vi "Settings Dialog.vi"(8 "error in (no error)":T5 caption="entrée d'erreur (pas d'erreur)", 11 "Paramètres en entrée":T1={"Configuration du matériel"={"Refnum de matériel <À remplacer>"="", "Type de signal <À remplacer>"=enum."Sine Wave", "Choix de la longueur d'onde"=500.0, "Nom du périphérique"="Dev1", "Choix mode"=FALSE}, "Configuration de l'enregistrement"={"Chemin de base du fichier journal"=path "", "Référence de fichier TDMS"=refnum}, "Commande numérique"=0.0}) -> (0 "error out":T5 caption="sortie d'erreur", 1 "Annulation ?":bool, 2 "Actualisation de l'IU requise ?":bool, 3 "Paramètres en sortie":T1={"Configuration du matériel"={"Refnum de matériel <À remplacer>"="", "Type de signal <À remplacer>"=enum."Sine Wave", "Choix de la longueur d'onde"=500.0, "Nom du périphérique"="Dev1", "Choix mode"=FALSE}, "Configuration de l'enregistrement"={"Chemin de base du fichier journal"=path "", "Référence de fichier TDMS"=refnum}, "Commande numérique"=0.0})   [LabVIEW 2018, in "Settings.lvlib"]
doc: "Boîte de dialogue permettant de sélectionner les paramètres spécifiés par l'utilisateur."
uses:
  Settings.lvlib
  Settings.ctl
  Acquisition/Hardware Configuration.ctl
  Acquisition/Signal Type.ctl
  Logging/Logging Configuration.ctl
  <vilib>/Utility/xml.llb/Write to XML File(string).vi
  Acquisition/Acquisition.lvlib
  Logging/Logging.lvlib
panel:
  in  "Nom du périphérique":tag="Dev1"
  in  "Choix de la longueur d'onde":dbl=500.0 min=500.0 max=2500.0 step=1.0
  in  "Choix mode":bool
  in  "Chemin du fichier journal":path
  in  "Type de signal":u16(ring) items=["Signal sinusoïdal", "Carré avec bruit", "Signal triangulaire", "Simulation DAQ"]
  in  "Bouton Annuler":bool
  in  "Bouton OK":bool
  # "Partie non visible de la boîte de dialogue (nécessaire au connecteur)."
  # "Mode manuel"
  # "Mode automatique"
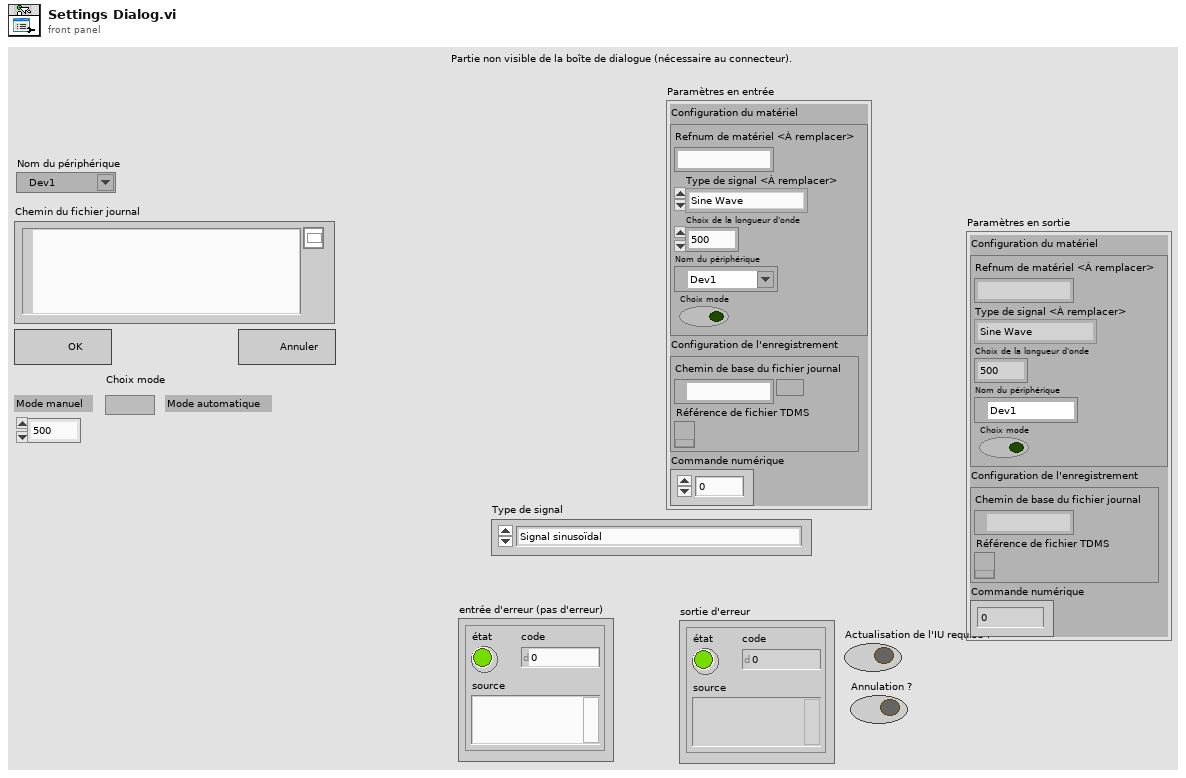
[diagram p1: front panel]
types:
  T1 = typedef "Settings.lvlib/Settings.ctl" = cluster{"Configuration du matériel":T2, "Configuration de l'enregistrement":T4, "Commande numérique":dbl}
  T2 = typedef "Acquisition.lvlib/Hardware Configuration.ctl" = cluster{"Refnum de matériel <À remplacer>":string, "Type de signal <À remplacer>":T3, "Choix de la longueur d'onde":dbl, "Nom du périphérique":tag, "Choix mode":bool}
  T3 = typedef "Acquisition.lvlib/Signal Type.ctl" = enum16{"Sine Wave", "Square with Noise", "Signal triangulaire", "Simulation DAQ"}
  T4 = typedef "Logging.lvlib/Logging Configuration.ctl" = cluster{"Chemin de base du fichier journal":path, "Référence de fichier TDMS":refnum<k34>}
  T5 = cluster{"état":bool, "code":i32, "source":string}
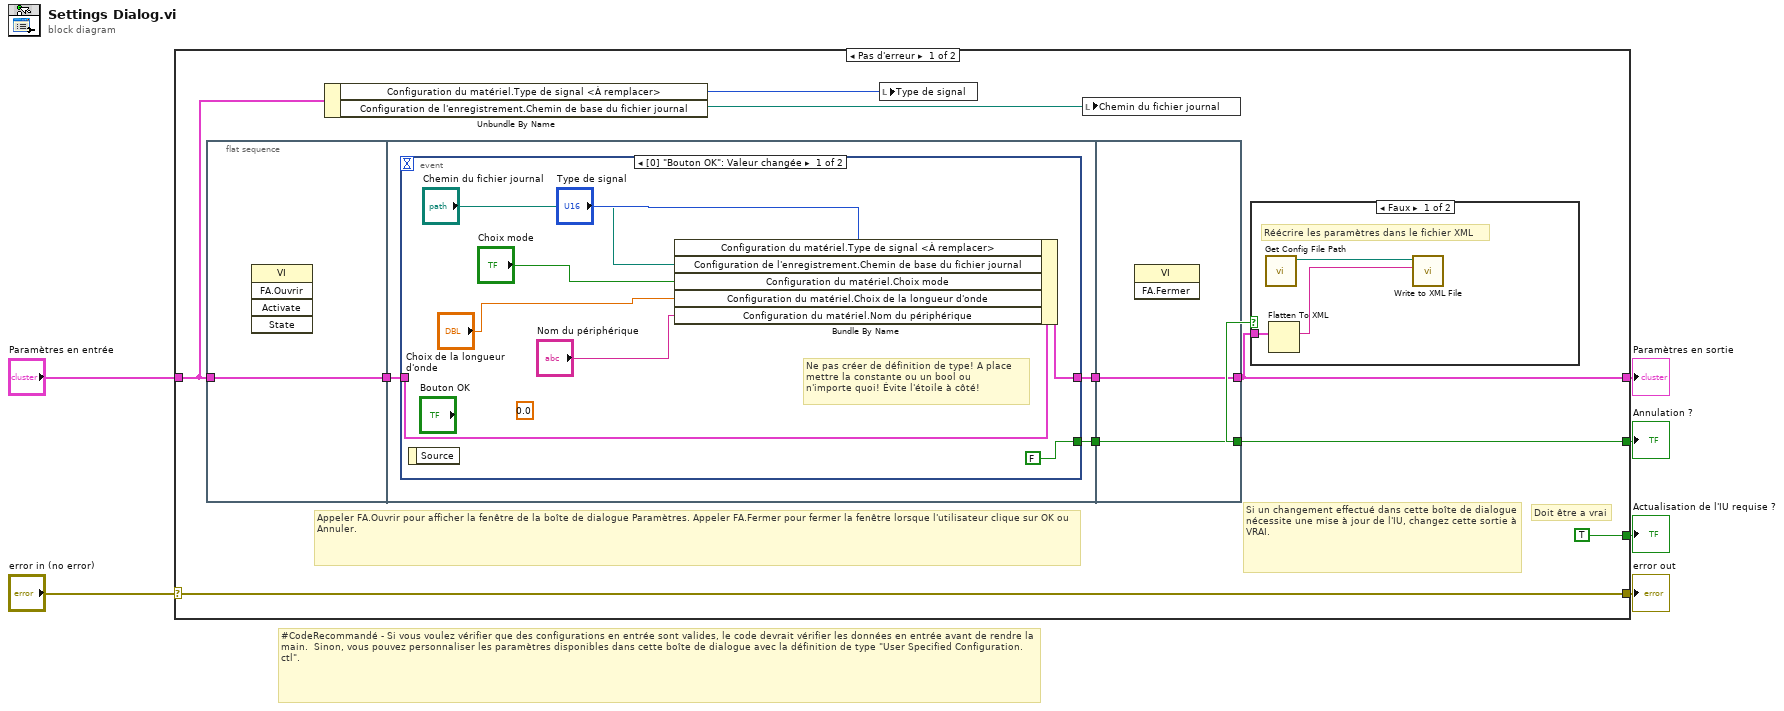
[diagram p0: block diagram]
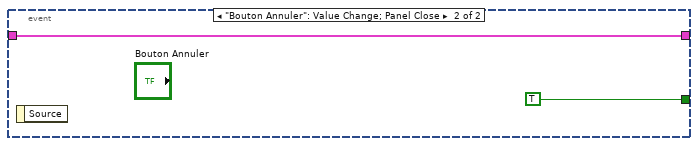
[diagram p2: hidden frame]
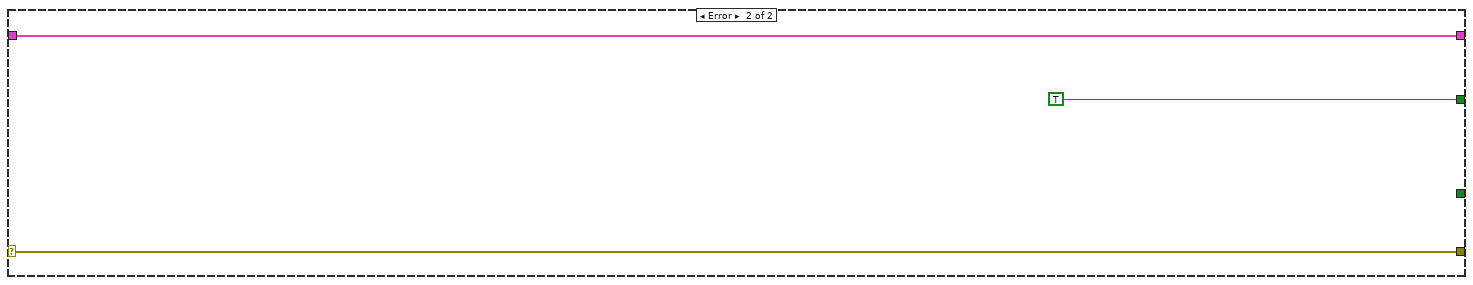
[diagram p4: hidden frame]
diagram:
  # "#CodeRecommandé - Si vous voulez vérifier que des configurations en entrée sont valides, le code devrait vérifier les données en entrée avant de rendre la main.  Sinon, vous pouvez personnaliser les paramètres disponibles dans cette boîte de dialogue avec la définition de type \"User Specified Configuration.ctl\"."
  n1 = case shown="Pas d'erreur" "error in (no error)" {
    selector: "error in (no error)" -> [w16 w38]
    tunnel: [w16 w38] -> w5
    tunnel: "Paramètres en entrée" -> [w12 w37]
    tunnel: [w13 w37] -> w3
    tunnel: [TRUE ("UI Refresh Needed?") _] -> w2
    tunnel: [w14 TRUE ("UI Refresh Needed?")] -> w1
    frame No Error {
      # "Doit être a vrai"
      # "Appeler FA.Ouvrir pour afficher la fenêtre de la boîte de dialogue Paramètres. Appeler FA.Fermer pour fermer la fenêtre lorsque l'utilisateur clique sur OK ou Annuler."
      # "Si un changement effectué dans cette boîte de dialogue nécessite une mise à jour de l'IU, changez cette sortie à VRAI."
      n2 = flat-sequence {
        tunnel: w12 -> [w17]
        tunnel: [w17] -> w9
        tunnel: w9 -> [w18]
        tunnel: [w20] -> w8
        tunnel: [w19] -> w7
        tunnel: [w31] -> w13
        tunnel: [w32] -> w14
        tunnel: w8 -> [w32]
        tunnel: w7 -> [w31]
        frame #0 {
          n3 = invoke class="VI" method="FA.Ouvrir"() -> ()  [unwired: 5 in, 5 out]
        }
        frame #1 {
          n4 = event shown="[0] \"Bouton OK\": Valeur changée" {
            selector: _ -> [_ _]
            dyn-events: _ -> [_ _]
            timeout: _ -> [_ _]
            tunnel: [w26 w30] -> w19
            tunnel: w18 -> [w27 w30]
            tunnel: [FALSE ("UI Refresh Needed?") TRUE ("UI Refresh Needed?")] -> w20
            event "Bouton OK": Value Change {
              (unwired) 0.0
              # "Ne pas créer de définition de type! A place\nmettre la constante ou un bool ou \nn'importe quoi! Évite l'étoile à côté!"
              n5 = event-data() -> ()  [unwired: 1 in, 1 out]
              n6 = Bundle By Name(cluster=w27, "Configuration du matériel.Type de signal <À remplacer>"="Type de signal", "Configuration de l'enregistrement.Chemin de base du fichier journal"="Chemin du fichier journal", "Configuration du matériel.Choix mode"="Choix mode", "Configuration du matériel.Choix de la longueur d'onde"="Choix de la longueur d'onde", "Configuration du matériel.Nom du périphérique"="Nom du périphérique") -> (w26:T1)
            }
            event "Bouton Annuler": Value Change; Panel Close {
              n7 = event-data() -> ()  [unwired: 1 in, 1 out]
            }
          }
        }
        frame #2 {
          n8 = invoke class="VI" method="FA.Fermer"() -> ()  [unwired: 3 in, 3 out]
        }
      }
      n9 = Unbundle By Name(w12) -> ("Configuration du matériel.Type de signal <À remplacer>"=w11:T3, "Configuration de l'enregistrement.Chemin de base du fichier journal"=w10:path)
      n10 = local write "Type de signal"(w11) -> ()
      n11 = local write "Chemin du fichier journal"(w10) -> ()
      n12 = case shown="Faux" w14 {
        tunnel: w13 -> [w34 _]
        frame False {
          # "Réécrire les paramètres dans le fichier XML"
          n13 = call "Get Config File Path.vi"() -> ("Chemin du fichier XML"=w35:path)  [unwired: 10 in, 1 out]
          n14 = Flatten To XML(anything=w34) -> (xml string=w33:string)
          n15 = call-poly <vilib>:"Write to XML File.vi"("XML Input"=w33, "XML File Path"=w35) -> ()  [unwired: 7 in, 3 out]
        }
        frame True {
        }
      }
    }
    frame Error {
    }
  }
  "Actualisation de l'IU requise ?" <- w2
  "error out" <- w5
  "Paramètres en sortie" <- w3
  "Annulation ?" <- w1
